vi "SetIntakeAngle.vi"(8 "error in (no error)":errorcluster, 9 "Angel(degrees)":dbl, 11 "Elevator Concrete in":refnum<class "Elevator Concrete.lvclass">) -> (0 "error out":errorcluster, 3 "Elevator Concrete out":refnum<class "Elevator Concrete.lvclass">)   [LabVIEW 2018]
uses:
  Elevator Concrete.lvclass
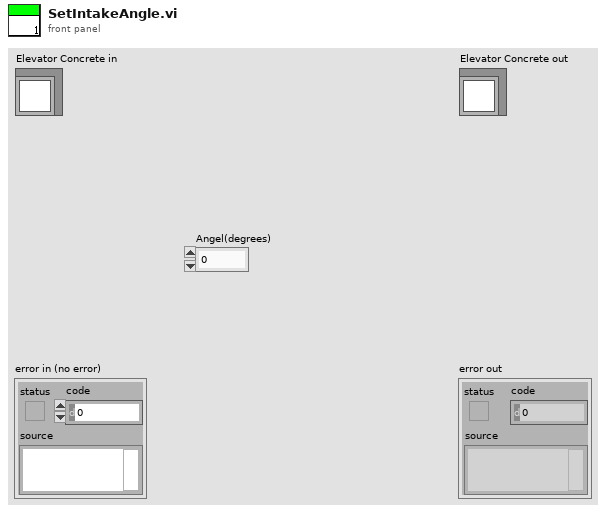
[diagram p1: front panel]
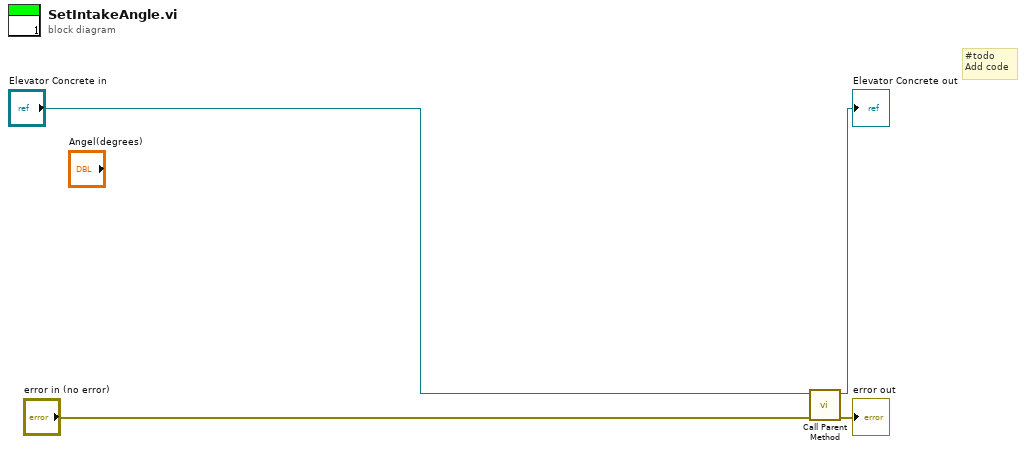
[diagram p0: block diagram]
diagram:
  # "#todo \nAdd code"
  n1 = call-parent "Call Parent Method"("error in (no error)"="error in (no error)", "Elevator in"="Elevator Concrete in") -> ("error out"=→"error out":errorcluster, "Elevator out"=→"Elevator Concrete out":refnum<class "Elevator Concrete.lvclass">)  [unwired: 8 in]
